vi "Dust_Type.vi"() -> ()   [LabVIEW 2013]
doc: "Searches the dust_type table for a user-selected dust name. For use in the Dust Lab. All results can be ordered by id_dust_type, dust name, density, source mass, bottle mass, or dust mass."
uses:
  Controls/Dust_list.ctl
  <vilib>/Utility/miscctls.llb/LVPointTypeDef.ctl
panel:
  in  "Update Type":bool
  out "Descending":string
  out "Ascending":string
  out "dust_weight text":string
  out "bottle_weight text":string
  out "source_weight text":string
  out "dust_density text":string
  out "dust_name text":string
  out "id_dust_type text":string
  in  "Exit":bool
  out "error out":errorcluster
  in  "error in (no error)":errorcluster
  in  "dust_weight":bool
  in  "bottle_weight":bool
  in  "source_weight":bool
  in  "dust_density":bool
  in  "dust_name":bool
  in  "id_dust_type":bool
  out "Array":T1[](array[typedef])
  # "Size"
  # "Comments"
  # "Shoots?"
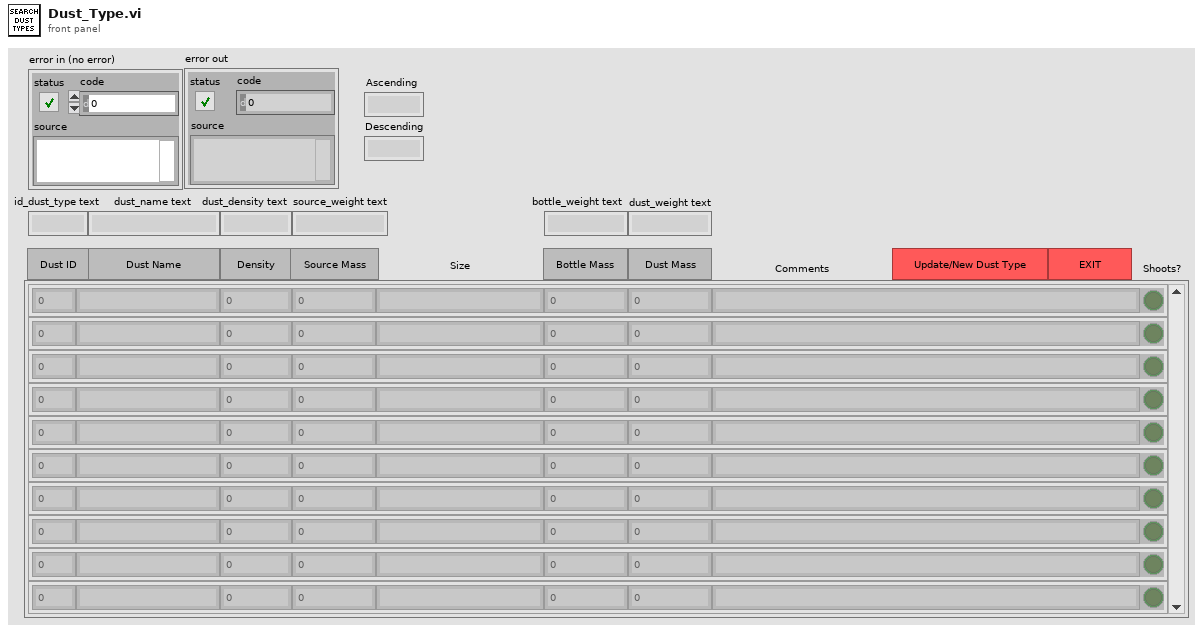
[diagram p1: front panel]
types:
  T1 = typedef "Dust_list.ctl" = cluster{"id_dust_type":i32, "dust_name":string, "dust_type":i32, "batch_no":i32, "dust_density":dbl, "source_weight":dbl, "size":string, "bottle_weight":dbl, "dust_mass":dbl, "comments":string, "Shoots?":bool}
  T2 = typedef "LVPointTypeDef.ctl" = cluster{"Horizontal":i16, "Vertical":i16}
  T3 = enum16{"dust_name", "dust_density", "source_weight", "bottle_weight", "dust_weight"}
  T4 = typedef "LVPoint32TypeDef.ctl" = cluster{"Horizontal":i32, "Vertical":i32}
  T5 = typedef "LVPositionTypeDef.ctl" = cluster{"Left":i32, "Top":i32}
  T6 = typedef "LVBoundsTypeDef.ctl" = cluster{"Width":u32, "Height":u32}
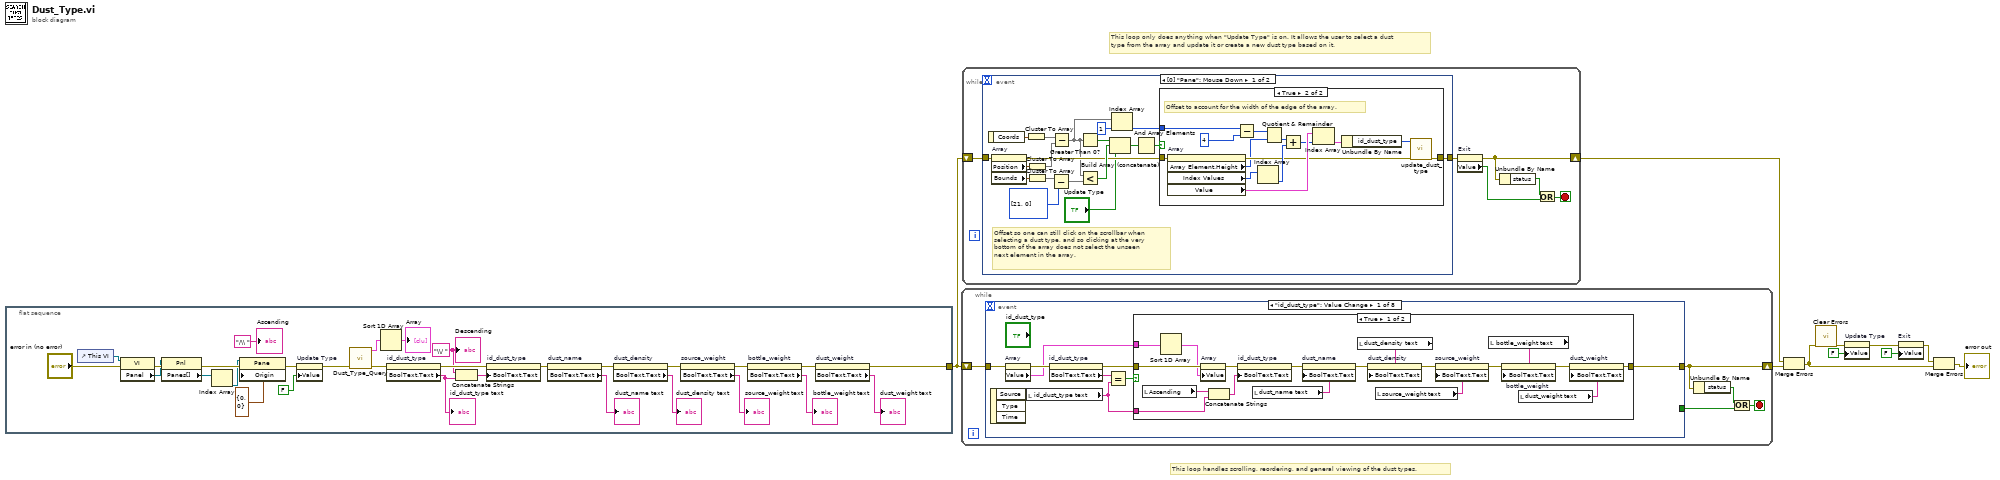
[diagram p0: block diagram]
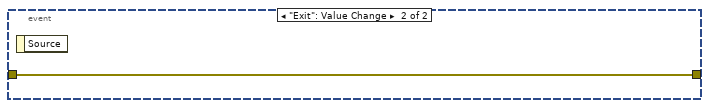
[diagram p3: hidden frame]
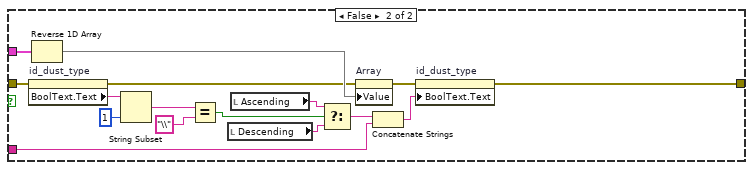
[diagram p4: hidden frame]
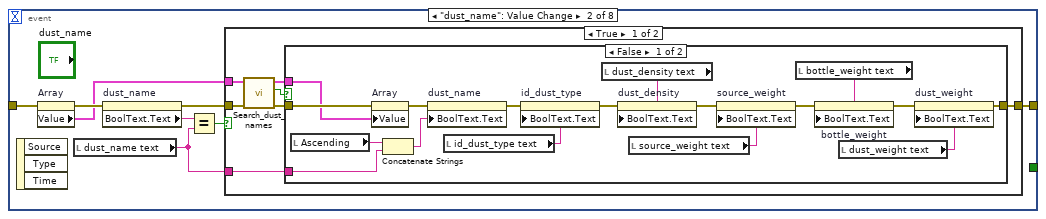
[diagram p5: hidden frame]
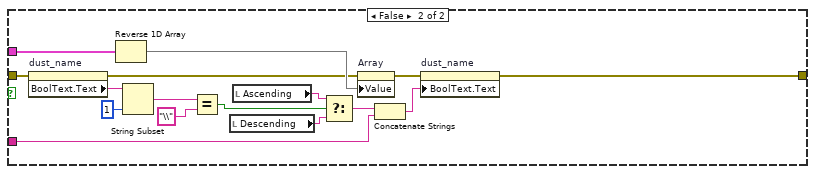
[diagram p7: hidden frame]
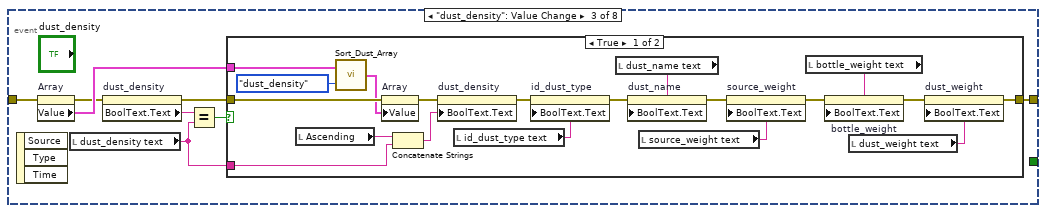
[diagram p8: hidden frame]
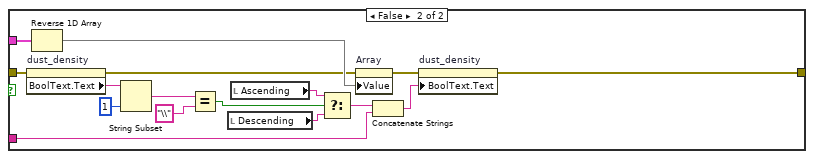
[diagram p9: hidden frame]
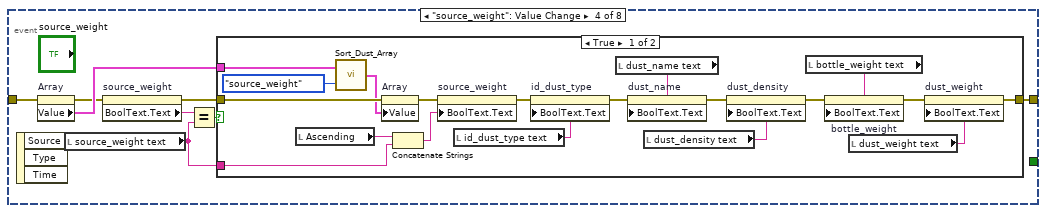
[diagram p10: hidden frame]
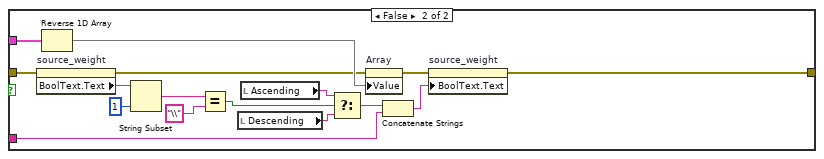
[diagram p11: hidden frame]
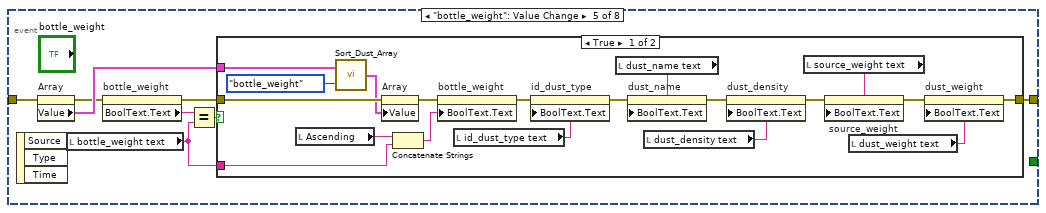
[diagram p12: hidden frame]
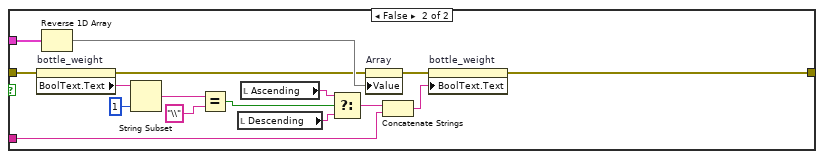
[diagram p13: hidden frame]
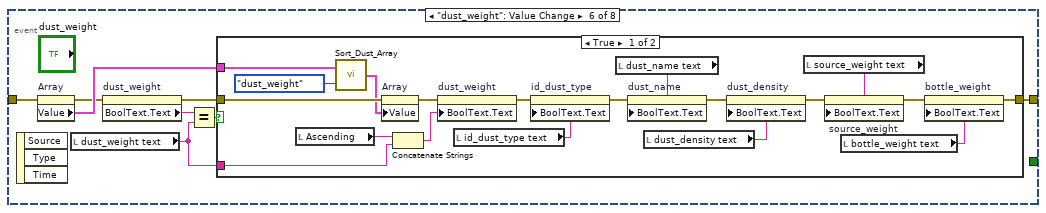
[diagram p14: hidden frame]
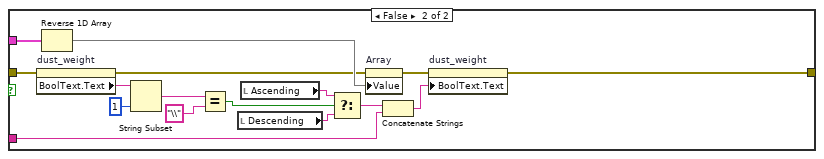
[diagram p15: hidden frame]
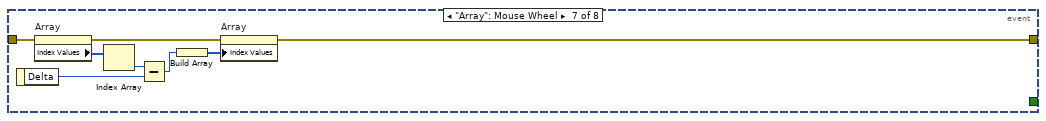
[diagram p16: hidden frame]
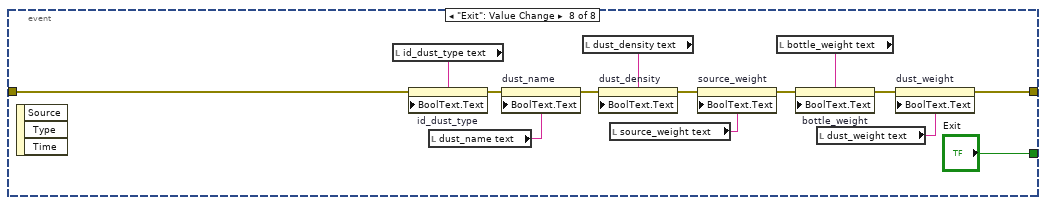
[diagram p17: hidden frame]
diagram:
  # "This loop handles scrolling, reordering, and general viewing of the dust types."
  # "This loop only does anything when \"Update Type\" is on. It allows the user to select a dust\ntype from the array and update it or create a new dust type based on it."
  n1 = flat-sequence {
    tunnel: [w31] -> w10
    frame #0 {
      w16 = "\\/ " ("Descending")
      n2 = control-ref of="This VI"() -> (w28:refnum<vi>)
      n3 = property class="VI"(reference=w28, error in="error in (no error)") -> (error out=w27:errorcluster, "Panel"=w26:refnum<vi>)  [unwired: 1 out]
      n4 = property class="Pnl"(reference=w26, error in=w27) -> (error out=w25:errorcluster, "Panes[]"=w24:refnum<vi>[])  [unwired: 1 out]
      n5 = Index Array(array=w24) -> (element=w23:refnum<vi>)  [unwired: 1 in]
      n6 = property class="Pane"(reference=w23, error in=w25, "Origin"=T2 {"Horizontal"=0, "Vertical"=0}) -> (error out=w13:errorcluster)  [unwired: 1 out]
      n7 = property on="Update Type" class="Bool (strict)"(error in=w13, "Value"=FALSE ("Update Type")) -> (error out=w12:errorcluster)  [unwired: 1 in, 1 out]
      n8 = call "Dust_Type_Query.vi"("error in (no error)"=w12) -> ("error out"=w30:errorcluster, "Dust Type Array"=w14:T1[])  [unwired: 9 in]
      n9 = Sort 1D Array(array=w14) -> (sorted array=→"Array":T1[])
      n10 = property on="id_dust_type" class="Bool"(error in=w30) -> (error out=w20:errorcluster, "BoolText.Text"=w18:string)  [unwired: 1 in, 1 out]
      "id_dust_type text" <- w18
      n11 = Concatenate Strings(w16, w18) -> (w19:string)
      n12 = property on="id_dust_type" class="Bool"(error in=w20, "BoolText.Text"=w19) -> (error out=w21:errorcluster)  [unwired: 1 in, 1 out]
      n13 = property on="dust_name" class="Bool"(error in=w21) -> (error out=w40:errorcluster, "BoolText.Text"=→"dust_name text":string)  [unwired: 1 in, 1 out]
      n14 = property on="dust_density" class="Bool"(error in=w40) -> (error out=w37:errorcluster, "BoolText.Text"=→"dust_density text":string)  [unwired: 1 in, 1 out]
      n15 = property on="source_weight" class="Bool"(error in=w37) -> (error out=w35:errorcluster, "BoolText.Text"=→"source_weight text":string)  [unwired: 1 in, 1 out]
      n16 = property on="bottle_weight" class="Bool"(error in=w35) -> (error out=w33:errorcluster, "BoolText.Text"=→"bottle_weight text":string)  [unwired: 1 in, 1 out]
      n17 = property on="dust_weight" class="Bool"(error in=w33) -> (error out=w31:errorcluster, "BoolText.Text"=→"dust_weight text":string)  [unwired: 1 in, 1 out]
      "Ascending" <- "/\\ " ("Ascending")
      "Descending" <- w16
    }
  }
  n18 = while {
    shift-right: [w41] -> w9
    shift-left: w10 -> [w45]
    stop <- w42 stop-if-true
    n19 = event shown="[0] \"id_dust_type\": Value Change" {
      selector: _ -> [_ _ _ _ _ _ _ _]
      dyn-events: _ -> [_ _ _ _ _ _ _ _]
      timeout: _ -> [_ _ _ _ _ _ _ _]
      tunnel: w45 -> [w53 w95 w144 w187 w230 w273 w314 w324]
      tunnel: [w52 w94 w143 w186 w229 w272 w309 w323] -> w41
      tunnel: [_ _ _ _ _ _ _ "Exit"] -> w44
      event "id_dust_type": Value Change {
        n20 = event-data() -> ()  [unwired: 1 in, 3 out]
        n21 = property on="Array" class="Arr (strict)"(error in=w53) -> (error out=w47:errorcluster, "Value"=w46:T1[])  [unwired: 1 in, 1 out]
        n22 = local read "id_dust_type text"() -> (w50:string)
        n23 = property on="id_dust_type" class="Bool"(error in=w47) -> (error out=w48:errorcluster, "BoolText.Text"=w51:string)  [unwired: 1 in, 1 out]
        n24 = Equal?(x=w51, y=w50) -> (x = y?=w49:bool)
        n25 = case shown="True" w49 {
          tunnel: [w58 w86] -> w52
          tunnel: w50 -> [w69 w85]
          tunnel: w48 -> [w57 w74]
          tunnel: w46 -> [w55 w84]
          frame True {
            n26 = local read "Ascending"() -> (w70:string)
            n27 = Sort 1D Array(array=w55) -> (sorted array=w54:T1[])
            n28 = property on="Array" class="Arr (strict)"(error in=w57, "Value"=w54) -> (error out=w56:errorcluster)  [unwired: 1 in, 1 out]
            n29 = Concatenate Strings(w70, w69) -> (w71:string)
            n30 = property on="id_dust_type" class="Bool"(error in=w56, "BoolText.Text"=w71) -> (error out=w59:errorcluster)  [unwired: 1 in, 1 out]
            n31 = local read "dust_name text"() -> (w63:string)
            n32 = property on="dust_name" class="Bool"(error in=w59, "BoolText.Text"=w63) -> (error out=w64:errorcluster)  [unwired: 1 in, 1 out]
            n33 = local read "dust_density text"() -> (w62:string)
            n34 = property on="dust_density" class="Bool"(error in=w64, "BoolText.Text"=w62) -> (error out=w65:errorcluster)  [unwired: 1 in, 1 out]
            n35 = local read "source_weight text"() -> (w61:string)
            n36 = property on="source_weight" class="Bool"(error in=w65, "BoolText.Text"=w61) -> (error out=w66:errorcluster)  [unwired: 1 in, 1 out]
            n37 = local read "bottle_weight text"() -> (w60:string)
            n38 = property on="bottle_weight" class="Bool"(error in=w66, "BoolText.Text"=w60) -> (error out=w67:errorcluster)  [unwired: 1 in, 1 out]
            n39 = local read "dust_weight text"() -> (w68:string)
            n40 = property on="dust_weight" class="Bool"(error in=w67, "BoolText.Text"=w68) -> (error out=w58:errorcluster)  [unwired: 1 in, 1 out]
          }
          frame False {
            n41 = property on="id_dust_type" class="Bool"(error in=w74) -> (error out=w73:errorcluster, "BoolText.Text"=w80:string)  [unwired: 1 in, 1 out]
            n42 = Reverse 1D Array(array=w84) -> (reversed array=w83:T1[])
            n43 = String Subset(string=w80, length (rest)=1 ("length (rest)")) -> (substring=w77:string)  [unwired: 1 in]
            n44 = Equal?(x=w77, y="\\") -> (x = y?=w75:bool)
            n45 = local read "Descending"() -> (w82:string)
            n46 = local read "Ascending"() -> (w78:string)
            n47 = Select(t=w78, s=w75, f=w82) -> (s? t:f=w81:string)
            n48 = property on="Array" class="Arr (strict)"(error in=w73, "Value"=w83) -> (error out=w72:errorcluster)  [unwired: 1 in, 1 out]
            n49 = Concatenate Strings(w81, w85) -> (w87:string)
            n50 = property on="id_dust_type" class="Bool"(error in=w72, "BoolText.Text"=w87) -> (error out=w86:errorcluster)  [unwired: 1 in, 1 out]
          }
        }
      }
      event "dust_name": Value Change {
        n51 = event-data() -> ()  [unwired: 1 in, 3 out]
        n52 = property on="Array" class="Arr (strict)"(error in=w95) -> (error out=w91:errorcluster, "Value"=w89:T1[])  [unwired: 1 in, 1 out]
        n53 = local read "dust_name text"() -> (w93:string)
        n54 = property on="dust_name" class="Bool"(error in=w91) -> (error out=w88:errorcluster, "BoolText.Text"=w90:string)  [unwired: 1 in, 1 out]
        n55 = Equal?(x=w90, y=w93) -> (x = y?=w92:bool)
        n56 = case shown="True" w92 {
          tunnel: [w101 w122] -> w94
          tunnel: w93 -> [w102 w136]
          tunnel: w88 -> [w100 w126]
          tunnel: w89 -> [w98 w135]
          frame True {
            n57 = call "Search_dust_names.vi"("error in (no error)"=w100, "Dust array in"=w98) -> ("error out"=w99:errorcluster, "Cancelled?"=w96:bool, "Dust array out"=w97:T1[])  [unwired: 7 in]
            n58 = case shown="False" w96 {
              tunnel: w102 -> [w118 _]
              tunnel: [w108 w120] -> w101
              tunnel: w99 -> [w104 w120]
              tunnel: w97 -> [w103 _]
              frame False {
                n59 = local read "Ascending"() -> (w119:string)
                n60 = property on="Array" class="Arr (strict)"(error in=w104, "Value"=w103) -> (error out=w106:errorcluster)  [unwired: 1 in, 1 out]
                n61 = Concatenate Strings(w119, w118) -> (w105:string)
                n62 = property on="dust_name" class="Bool"(error in=w106, "BoolText.Text"=w105) -> (error out=w107:errorcluster)  [unwired: 1 in, 1 out]
                n63 = local read "id_dust_type text"() -> (w112:string)
                n64 = property on="id_dust_type" class="Bool"(error in=w107, "BoolText.Text"=w112) -> (error out=w113:errorcluster)  [unwired: 1 in, 1 out]
                n65 = local read "dust_density text"() -> (w111:string)
                n66 = property on="dust_density" class="Bool"(error in=w113, "BoolText.Text"=w111) -> (error out=w114:errorcluster)  [unwired: 1 in, 1 out]
                n67 = local read "source_weight text"() -> (w110:string)
                n68 = property on="source_weight" class="Bool"(error in=w114, "BoolText.Text"=w110) -> (error out=w115:errorcluster)  [unwired: 1 in, 1 out]
                n69 = local read "bottle_weight text"() -> (w109:string)
                n70 = property on="bottle_weight" class="Bool"(error in=w115, "BoolText.Text"=w109) -> (error out=w116:errorcluster)  [unwired: 1 in, 1 out]
                n71 = local read "dust_weight text"() -> (w117:string)
                n72 = property on="dust_weight" class="Bool"(error in=w116, "BoolText.Text"=w117) -> (error out=w108:errorcluster)  [unwired: 1 in, 1 out]
              }
              frame True {
              }
            }
          }
          frame False {
            n73 = property on="dust_name" class="Bool"(error in=w126) -> (error out=w125:errorcluster, "BoolText.Text"=w124:string)  [unwired: 1 in, 1 out]
            n74 = Reverse 1D Array(array=w135) -> (reversed array=w134:T1[])
            n75 = String Subset(string=w124, length (rest)=1 ("length (rest)")) -> (substring=w129:string)  [unwired: 1 in]
            n76 = Equal?(x=w129, y="\\") -> (x = y?=w127:bool)
            n77 = local read "Descending"() -> (w133:string)
            n78 = local read "Ascending"() -> (w130:string)
            n79 = Select(t=w130, s=w127, f=w133) -> (s? t:f=w132:string)
            n80 = property on="Array" class="Arr (strict)"(error in=w125, "Value"=w134) -> (error out=w123:errorcluster)  [unwired: 1 in, 1 out]
            n81 = Concatenate Strings(w132, w136) -> (w121:string)
            n82 = property on="dust_name" class="Bool"(error in=w123, "BoolText.Text"=w121) -> (error out=w122:errorcluster)  [unwired: 1 in, 1 out]
          }
        }
      }
      event "dust_density": Value Change {
        n83 = event-data() -> ()  [unwired: 1 in, 3 out]
        n84 = property on="Array" class="Arr (strict)"(error in=w144) -> (error out=w139:errorcluster, "Value"=w140:T1[])  [unwired: 1 in, 1 out]
        n85 = local read "dust_density text"() -> (w142:string)
        n86 = property on="dust_density" class="Bool"(error in=w139) -> (error out=w137:errorcluster, "BoolText.Text"=w138:string)  [unwired: 1 in, 1 out]
        n87 = Equal?(x=w138, y=w142) -> (x = y?=w141:bool)
        n88 = case shown="True" w141 {
          tunnel: [w152 w165] -> w143
          tunnel: w142 -> [w162 w179]
          tunnel: w137 -> [w151 w169]
          tunnel: w140 -> [w150 w178]
          frame True {
            n89 = local read "Ascending"() -> (w163:string)
            n90 = call "Sort_Dust_Array.vi"("Order by..."=T3."dust_density", "Array In"=w150) -> ("Array out"=w149:T1[])
            n91 = property on="Array" class="Arr (strict)"(error in=w151, "Value"=w149) -> (error out=w147:errorcluster)  [unwired: 1 in, 1 out]
            n92 = Concatenate Strings(w163, w162) -> (w146:string)
            n93 = property on="dust_density" class="Bool"(error in=w147, "BoolText.Text"=w146) -> (error out=w148:errorcluster)  [unwired: 1 in, 1 out]
            n94 = local read "id_dust_type text"() -> (w156:string)
            n95 = property on="id_dust_type" class="Bool"(error in=w148, "BoolText.Text"=w156) -> (error out=w157:errorcluster)  [unwired: 1 in, 1 out]
            n96 = local read "dust_name text"() -> (w155:string)
            n97 = property on="dust_name" class="Bool"(error in=w157, "BoolText.Text"=w155) -> (error out=w158:errorcluster)  [unwired: 1 in, 1 out]
            n98 = local read "source_weight text"() -> (w154:string)
            n99 = property on="source_weight" class="Bool"(error in=w158, "BoolText.Text"=w154) -> (error out=w159:errorcluster)  [unwired: 1 in, 1 out]
            n100 = local read "bottle_weight text"() -> (w153:string)
            n101 = property on="bottle_weight" class="Bool"(error in=w159, "BoolText.Text"=w153) -> (error out=w160:errorcluster)  [unwired: 1 in, 1 out]
            n102 = local read "dust_weight text"() -> (w161:string)
            n103 = property on="dust_weight" class="Bool"(error in=w160, "BoolText.Text"=w161) -> (error out=w152:errorcluster)  [unwired: 1 in, 1 out]
          }
          frame False {
            n104 = property on="dust_density" class="Bool"(error in=w169) -> (error out=w168:errorcluster, "BoolText.Text"=w167:string)  [unwired: 1 in, 1 out]
            n105 = Reverse 1D Array(array=w178) -> (reversed array=w177:T1[])
            n106 = String Subset(string=w167, length (rest)=1 ("length (rest)")) -> (substring=w172:string)  [unwired: 1 in]
            n107 = Equal?(x=w172, y="\\") -> (x = y?=w170:bool)
            n108 = local read "Descending"() -> (w176:string)
            n109 = local read "Ascending"() -> (w173:string)
            n110 = Select(t=w173, s=w170, f=w176) -> (s? t:f=w175:string)
            n111 = property on="Array" class="Arr (strict)"(error in=w168, "Value"=w177) -> (error out=w166:errorcluster)  [unwired: 1 in, 1 out]
            n112 = Concatenate Strings(w175, w179) -> (w164:string)
            n113 = property on="dust_density" class="Bool"(error in=w166, "BoolText.Text"=w164) -> (error out=w165:errorcluster)  [unwired: 1 in, 1 out]
          }
        }
      }
      event "source_weight": Value Change {
        n114 = event-data() -> ()  [unwired: 1 in, 3 out]
        n115 = property on="Array" class="Arr (strict)"(error in=w187) -> (error out=w182:errorcluster, "Value"=w183:T1[])  [unwired: 1 in, 1 out]
        n116 = local read "source_weight text"() -> (w185:string)
        n117 = property on="source_weight" class="Bool"(error in=w182) -> (error out=w180:errorcluster, "BoolText.Text"=w181:string)  [unwired: 1 in, 1 out]
        n118 = Equal?(x=w181, y=w185) -> (x = y?=w184:bool)
        n119 = case shown="True" w184 {
          tunnel: [w195 w208] -> w186
          tunnel: w185 -> [w205 w222]
          tunnel: w180 -> [w194 w212]
          tunnel: w183 -> [w193 w221]
          frame True {
            n120 = local read "Ascending"() -> (w206:string)
            n121 = call "Sort_Dust_Array.vi"("Order by..."=T3."source_weight", "Array In"=w193) -> ("Array out"=w192:T1[])
            n122 = property on="Array" class="Arr (strict)"(error in=w194, "Value"=w192) -> (error out=w190:errorcluster)  [unwired: 1 in, 1 out]
            n123 = Concatenate Strings(w206, w205) -> (w189:string)
            n124 = property on="source_weight" class="Bool"(error in=w190, "BoolText.Text"=w189) -> (error out=w191:errorcluster)  [unwired: 1 in, 1 out]
            n125 = local read "id_dust_type text"() -> (w199:string)
            n126 = property on="id_dust_type" class="Bool"(error in=w191, "BoolText.Text"=w199) -> (error out=w200:errorcluster)  [unwired: 1 in, 1 out]
            n127 = local read "dust_name text"() -> (w198:string)
            n128 = property on="dust_name" class="Bool"(error in=w200, "BoolText.Text"=w198) -> (error out=w201:errorcluster)  [unwired: 1 in, 1 out]
            n129 = local read "dust_density text"() -> (w197:string)
            n130 = property on="dust_density" class="Bool"(error in=w201, "BoolText.Text"=w197) -> (error out=w202:errorcluster)  [unwired: 1 in, 1 out]
            n131 = local read "bottle_weight text"() -> (w196:string)
            n132 = property on="bottle_weight" class="Bool"(error in=w202, "BoolText.Text"=w196) -> (error out=w203:errorcluster)  [unwired: 1 in, 1 out]
            n133 = local read "dust_weight text"() -> (w204:string)
            n134 = property on="dust_weight" class="Bool"(error in=w203, "BoolText.Text"=w204) -> (error out=w195:errorcluster)  [unwired: 1 in, 1 out]
          }
          frame False {
            n135 = property on="source_weight" class="Bool"(error in=w212) -> (error out=w211:errorcluster, "BoolText.Text"=w210:string)  [unwired: 1 in, 1 out]
            n136 = Reverse 1D Array(array=w221) -> (reversed array=w220:T1[])
            n137 = String Subset(string=w210, length (rest)=1 ("length (rest)")) -> (substring=w215:string)  [unwired: 1 in]
            n138 = Equal?(x=w215, y="\\") -> (x = y?=w213:bool)
            n139 = local read "Descending"() -> (w219:string)
            n140 = local read "Ascending"() -> (w216:string)
            n141 = Select(t=w216, s=w213, f=w219) -> (s? t:f=w218:string)
            n142 = property on="Array" class="Arr (strict)"(error in=w211, "Value"=w220) -> (error out=w209:errorcluster)  [unwired: 1 in, 1 out]
            n143 = Concatenate Strings(w218, w222) -> (w207:string)
            n144 = property on="source_weight" class="Bool"(error in=w209, "BoolText.Text"=w207) -> (error out=w208:errorcluster)  [unwired: 1 in, 1 out]
          }
        }
      }
      event "bottle_weight": Value Change {
        n145 = event-data() -> ()  [unwired: 1 in, 3 out]
        n146 = property on="Array" class="Arr (strict)"(error in=w230) -> (error out=w225:errorcluster, "Value"=w226:T1[])  [unwired: 1 in, 1 out]
        n147 = local read "bottle_weight text"() -> (w228:string)
        n148 = property on="bottle_weight" class="Bool"(error in=w225) -> (error out=w223:errorcluster, "BoolText.Text"=w224:string)  [unwired: 1 in, 1 out]
        n149 = Equal?(x=w224, y=w228) -> (x = y?=w227:bool)
        n150 = case shown="True" w227 {
          tunnel: [w238 w251] -> w229
          tunnel: w228 -> [w248 w265]
          tunnel: w223 -> [w237 w255]
          tunnel: w226 -> [w236 w264]
          frame True {
            n151 = local read "Ascending"() -> (w249:string)
            n152 = call "Sort_Dust_Array.vi"("Order by..."=T3."bottle_weight", "Array In"=w236) -> ("Array out"=w235:T1[])
            n153 = property on="Array" class="Arr (strict)"(error in=w237, "Value"=w235) -> (error out=w233:errorcluster)  [unwired: 1 in, 1 out]
            n154 = Concatenate Strings(w249, w248) -> (w232:string)
            n155 = property on="bottle_weight" class="Bool"(error in=w233, "BoolText.Text"=w232) -> (error out=w234:errorcluster)  [unwired: 1 in, 1 out]
            n156 = local read "id_dust_type text"() -> (w242:string)
            n157 = property on="id_dust_type" class="Bool"(error in=w234, "BoolText.Text"=w242) -> (error out=w243:errorcluster)  [unwired: 1 in, 1 out]
            n158 = local read "dust_name text"() -> (w241:string)
            n159 = property on="dust_name" class="Bool"(error in=w243, "BoolText.Text"=w241) -> (error out=w244:errorcluster)  [unwired: 1 in, 1 out]
            n160 = local read "dust_density text"() -> (w240:string)
            n161 = property on="dust_density" class="Bool"(error in=w244, "BoolText.Text"=w240) -> (error out=w245:errorcluster)  [unwired: 1 in, 1 out]
            n162 = local read "source_weight text"() -> (w239:string)
            n163 = property on="source_weight" class="Bool"(error in=w245, "BoolText.Text"=w239) -> (error out=w246:errorcluster)  [unwired: 1 in, 1 out]
            n164 = local read "dust_weight text"() -> (w247:string)
            n165 = property on="dust_weight" class="Bool"(error in=w246, "BoolText.Text"=w247) -> (error out=w238:errorcluster)  [unwired: 1 in, 1 out]
          }
          frame False {
            n166 = property on="bottle_weight" class="Bool"(error in=w255) -> (error out=w254:errorcluster, "BoolText.Text"=w253:string)  [unwired: 1 in, 1 out]
            n167 = Reverse 1D Array(array=w264) -> (reversed array=w263:T1[])
            n168 = String Subset(string=w253, length (rest)=1 ("length (rest)")) -> (substring=w258:string)  [unwired: 1 in]
            n169 = Equal?(x=w258, y="\\") -> (x = y?=w256:bool)
            n170 = local read "Descending"() -> (w262:string)
            n171 = local read "Ascending"() -> (w259:string)
            n172 = Select(t=w259, s=w256, f=w262) -> (s? t:f=w261:string)
            n173 = property on="Array" class="Arr (strict)"(error in=w254, "Value"=w263) -> (error out=w252:errorcluster)  [unwired: 1 in, 1 out]
            n174 = Concatenate Strings(w261, w265) -> (w250:string)
            n175 = property on="bottle_weight" class="Bool"(error in=w252, "BoolText.Text"=w250) -> (error out=w251:errorcluster)  [unwired: 1 in, 1 out]
          }
        }
      }
      event "dust_weight": Value Change {
        n176 = event-data() -> ()  [unwired: 1 in, 3 out]
        n177 = property on="Array" class="Arr (strict)"(error in=w273) -> (error out=w268:errorcluster, "Value"=w269:T1[])  [unwired: 1 in, 1 out]
        n178 = local read "dust_weight text"() -> (w271:string)
        n179 = property on="dust_weight" class="Bool"(error in=w268) -> (error out=w266:errorcluster, "BoolText.Text"=w267:string)  [unwired: 1 in, 1 out]
        n180 = Equal?(x=w267, y=w271) -> (x = y?=w270:bool)
        n181 = case shown="True" w270 {
          tunnel: [w281 w294] -> w272
          tunnel: w271 -> [w291 w308]
          tunnel: w266 -> [w280 w298]
          tunnel: w269 -> [w279 w307]
          frame True {
            n182 = local read "Ascending"() -> (w292:string)
            n183 = call "Sort_Dust_Array.vi"("Order by..."=T3."dust_weight", "Array In"=w279) -> ("Array out"=w278:T1[])
            n184 = property on="Array" class="Arr (strict)"(error in=w280, "Value"=w278) -> (error out=w276:errorcluster)  [unwired: 1 in, 1 out]
            n185 = Concatenate Strings(w292, w291) -> (w275:string)
            n186 = property on="dust_weight" class="Bool"(error in=w276, "BoolText.Text"=w275) -> (error out=w277:errorcluster)  [unwired: 1 in, 1 out]
            n187 = local read "id_dust_type text"() -> (w285:string)
            n188 = property on="id_dust_type" class="Bool"(error in=w277, "BoolText.Text"=w285) -> (error out=w286:errorcluster)  [unwired: 1 in, 1 out]
            n189 = local read "dust_name text"() -> (w284:string)
            n190 = property on="dust_name" class="Bool"(error in=w286, "BoolText.Text"=w284) -> (error out=w287:errorcluster)  [unwired: 1 in, 1 out]
            n191 = local read "dust_density text"() -> (w283:string)
            n192 = property on="dust_density" class="Bool"(error in=w287, "BoolText.Text"=w283) -> (error out=w288:errorcluster)  [unwired: 1 in, 1 out]
            n193 = local read "source_weight text"() -> (w282:string)
            n194 = property on="source_weight" class="Bool"(error in=w288, "BoolText.Text"=w282) -> (error out=w289:errorcluster)  [unwired: 1 in, 1 out]
            n195 = local read "bottle_weight text"() -> (w290:string)
            n196 = property on="bottle_weight" class="Bool"(error in=w289, "BoolText.Text"=w290) -> (error out=w281:errorcluster)  [unwired: 1 in, 1 out]
          }
          frame False {
            n197 = property on="dust_weight" class="Bool"(error in=w298) -> (error out=w297:errorcluster, "BoolText.Text"=w296:string)  [unwired: 1 in, 1 out]
            n198 = Reverse 1D Array(array=w307) -> (reversed array=w306:T1[])
            n199 = String Subset(string=w296, length (rest)=1 ("length (rest)")) -> (substring=w301:string)  [unwired: 1 in]
            n200 = Equal?(x=w301, y="\\") -> (x = y?=w299:bool)
            n201 = local read "Descending"() -> (w305:string)
            n202 = local read "Ascending"() -> (w302:string)
            n203 = Select(t=w302, s=w299, f=w305) -> (s? t:f=w304:string)
            n204 = property on="Array" class="Arr (strict)"(error in=w297, "Value"=w306) -> (error out=w295:errorcluster)  [unwired: 1 in, 1 out]
            n205 = Concatenate Strings(w304, w308) -> (w293:string)
            n206 = property on="dust_weight" class="Bool"(error in=w295, "BoolText.Text"=w293) -> (error out=w294:errorcluster)  [unwired: 1 in, 1 out]
          }
        }
      }
      event "Array": Mouse Wheel {
        n207 = event-data() -> ("Delta"=w312:i32)  [unwired: 1 in]
        n208 = property on="Array" class="Arr (strict)"(error in=w314) -> (error out=w310:errorcluster, "Index Values"=w313:u32[])  [unwired: 1 in, 1 out]
        n209 = Index Array(array=w313) -> (element=w315:u32)  [unwired: 1 in]
        n210 = Subtract(x=w315, y=w312) -> (x-y=w316:u32)
        n211 = Build Array(w316) -> (w311:u32[])
        n212 = property on="Array" class="Arr (strict)"(error in=w310, "Index Values"=w311) -> (error out=w309:errorcluster)  [unwired: 1 in, 1 out]
      }
      event "Exit": Value Change {
        n213 = event-data() -> ()  [unwired: 1 in, 3 out]
        n214 = local read "id_dust_type text"() -> (w322:string)
        n215 = property on="id_dust_type" class="Bool"(error in=w324, "BoolText.Text"=w322) -> (error out=w325:errorcluster)  [unwired: 1 in, 1 out]
        n216 = local read "dust_name text"() -> (w321:string)
        n217 = property on="dust_name" class="Bool"(error in=w325, "BoolText.Text"=w321) -> (error out=w326:errorcluster)  [unwired: 1 in, 1 out]
        n218 = local read "dust_density text"() -> (w320:string)
        n219 = property on="dust_density" class="Bool"(error in=w326, "BoolText.Text"=w320) -> (error out=w327:errorcluster)  [unwired: 1 in, 1 out]
        n220 = local read "source_weight text"() -> (w319:string)
        n221 = property on="source_weight" class="Bool"(error in=w327, "BoolText.Text"=w319) -> (error out=w328:errorcluster)  [unwired: 1 in, 1 out]
        n222 = local read "bottle_weight text"() -> (w318:string)
        n223 = property on="bottle_weight" class="Bool"(error in=w328, "BoolText.Text"=w318) -> (error out=w329:errorcluster)  [unwired: 1 in, 1 out]
        n224 = local read "dust_weight text"() -> (w317:string)
        n225 = property on="dust_weight" class="Bool"(error in=w329, "BoolText.Text"=w317) -> (error out=w323:errorcluster)  [unwired: 1 in, 1 out]
      }
    }
    n226 = Unbundle By Name(w41) -> ("status"=w43:bool)
    n227 = Or(x=w43, y=w44) -> (x .or. y?=w42:bool)
  }
  n228 = while {
    shift-right: [w332] -> w8
    shift-left: w10 -> [w331]
    stop <- w335 stop-if-true
    n229 = event shown="[0] \"Pane\": Mouse Down" {
      selector: _ -> [_ _]
      dyn-events: _ -> [_ _]
      timeout: _ -> [_ _]
      tunnel: w331 -> [w346 w371]
      tunnel: [w340 w371] -> w333
      event Mouse Down {
        # "Offset so one can still click on the scrollbar when\nselecting a dust type, and so clicking at the very\nbottom of the array does not select the unseen\nnext element in the array."
        n230 = event-data() -> ("Coords"=w355:T4)  [unwired: 1 in]
        n231 = property on="Array" class="Arr (strict)"(error in=w346) -> (error out=w344:errorcluster, "Position"=w354:T5, "Bounds"=w351:T6)  [unwired: 1 in, 1 out]
        n232 = Cluster To Array(cluster=w355) -> (array=w353:i32[])
        n233 = Cluster To Array(cluster=w354) -> (array=w352:i32[])
        n234 = Cluster To Array(cluster=w351) -> (array=w350:u32[])
        n235 = Subtract(x=w350, y=u32[] [21, 0]) -> (x-y=w338:u32[])
        n236 = Subtract(x=w353, y=w352) -> (x-y=w343:i32[])
        n237 = Greater Than 0?(x=w343) -> (x > 0?=w349:bool[])
        n238 = Less?(x=w343, y=w338) -> (x < y?=w348:bool[])
        n239 = Build Array (concatenate)(w349, w348, "Update Type") -> (w347:bool[])
        n240 = Index Array(array=w343, index=1) -> (element=w341:i32)
        n241 = And Array Elements(Boolean array=w347) -> (logical AND=w345:bool)
        n242 = case shown="True" w345 {
          tunnel: [w356 w370] -> w340
          tunnel: w344 -> [w356 w369]
          tunnel: w341 -> [_ w358]
          frame False {
          }
          frame True {
            # "Offset to account for the width of the edge of the array."
            n243 = property on="Array" class="Arr (strict)"(error in=w369) -> (error out=w362:errorcluster, "Array Element.Height"=w360:u32, "Index Values"=w368:u32[], "Value"=w365:T1[])  [unwired: 1 in, 1 out]
            n244 = Subtract(x=w358, y=4) -> (x-y=w359:i32)
            n245 = Index Array(array=w368) -> (element=w366:u32)  [unwired: 1 in]
            n246 = Quotient & Remainder(x=w359, y=w360) -> (floor(x/y)=w367:u32)  [unwired: 1 out]
            n247 = Add(x=w367, y=w366) -> (x+y=w364:u32)
            n248 = Index Array(array=w365, index=w364) -> (element=w363:T1)
            n249 = Unbundle By Name(w363) -> ("id_dust_type"=w361:i32)
            n250 = call "update_dust_type.vi"("error in (no error)"=w362, "ID Dust Type"=w361) -> ("error out"=w370:errorcluster)  [unwired: 9 in]
          }
        }
      }
      event "Exit": Value Change {
        n251 = event-data() -> ()  [unwired: 1 in, 1 out]
      }
    }
    n252 = property on="Exit" class="Bool (strict)"(error in=w333) -> (error out=w332:errorcluster, "Value"=w334:bool)  [unwired: 1 in, 1 out]
    n253 = Unbundle By Name(w332) -> ("status"=w336:bool)
    n254 = Or(x=w336, y=w334) -> (x .or. y?=w335:bool)
  }
  n255 = Merge Errors(w8, w9) -> (w7:errorcluster)
  n256 = call <vilib>:"Clear Errors.vi"("error in (no error)"=w7) -> ("error out"=w3:errorcluster)  [unwired: 6 in]
  n257 = property on="Update Type" class="Bool (strict)"(error in=w3, "Value"=FALSE ("Update Type")) -> (error out=w1:errorcluster)  [unwired: 1 in, 1 out]
  n258 = property on="Exit" class="Bool (strict)"(error in=w1, "Value"=FALSE ("Value (Signaling)")) -> (error out=w4:errorcluster)  [unwired: 1 in, 1 out]
  n259 = Merge Errors(w4, w7) -> (→"error out":errorcluster)
